vi "Practica_1.vi"() -> ()   [LabVIEW 2020]
panel:
  out "Waveform Chart 2":dbl[](graph)
  out "Frecuencia":dbl format="%#_13g"
  out "Waveform Chart":dynamicdata(graph)
  in  "stop":bool
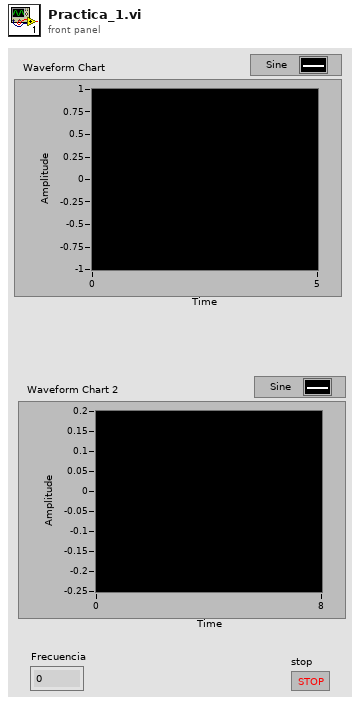
[diagram p1: front panel]
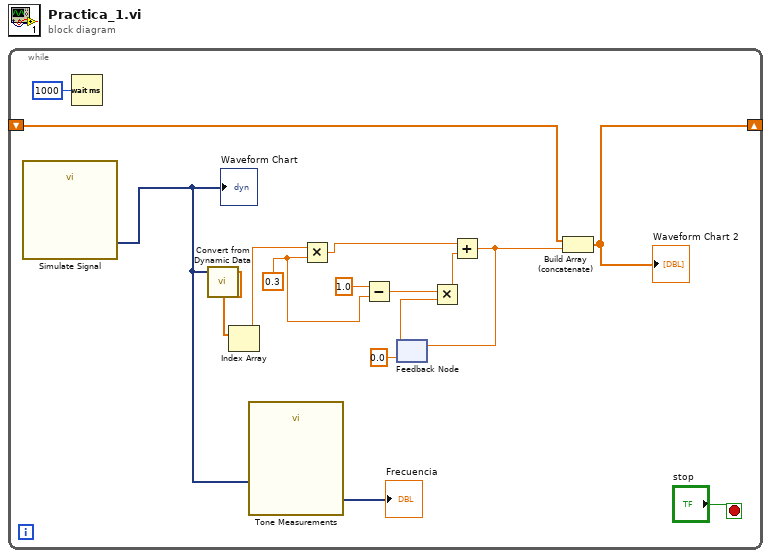
[diagram p0: block diagram]
diagram:
  n1 = while {
    shift-right: [w2] -> _
    shift-left: _ -> [w3]
    stop <- "stop" stop-if-true
    w14 = 0.3 ("y")
    n2 = call "Simulate Signal"() -> ("Sine"=w7:dynamicdata)  [unwired: 14 in, 1 out]
    "Waveform Chart" <- w7
    n3 = Wait (ms)(milliseconds to wait=u32 1000) -> ()  [unwired: 1 out]
    n4 = call "Convert from Dynamic Data"("Dynamic Data Type"=w7) -> ("Array"=w6:dbl[])  [unwired: 3 in]
    n5 = Index Array(array=w6) -> (element=w5:dbl)  [unwired: 1 in]
    n6 = call "Tone Measurements"("Signals"=w7) -> ("Frequency"=→"Frecuencia":dynamicdata)  [unwired: 9 in, 1 out]
    n7 = Multiply(x=w5, y=w14) -> (x*y=w10:dbl)
    n8 = Subtract(x=1.0, y=w14) -> (x-y=w12:dbl)
    n9 = feedback #1(0.0) -> (w9:dbl)
    n10 = Multiply(x=w12, y=w9) -> (x*y=w11:dbl)
    n11 = Add(x=w10, y=w11) -> (x+y=w4:dbl)
    n12 = feedback-in #1(w4) -> ()
    n13 = Build Array (concatenate)(w3, w4) -> (w2:dbl[])
    "Waveform Chart 2" <- w2
  }
